vi "Is Case Selector.vi"(8 "error in":errorcluster, 11 "Terminal in":refnum<vi>) -> (0 "error out":errorcluster, 3 "Is Case Selector":bool)   [LabVIEW 2023]
doc: "Returns True is case selector is of cluaster type (as in Error Cluster)."
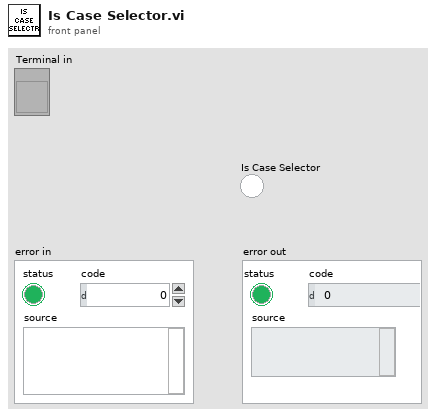
[diagram p1: front panel]
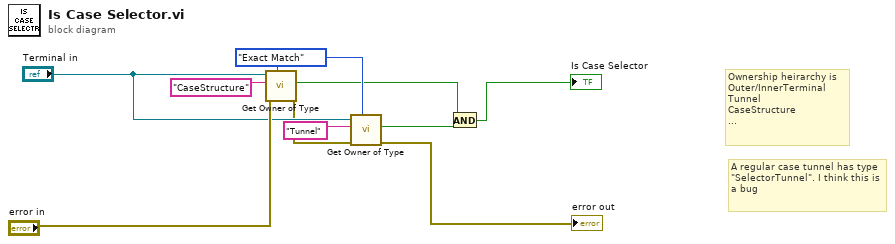
[diagram p0: block diagram]
diagram:
  w6 = enum16{"Exact Match", "Contains"}."Exact Match" ("Match Type")
  # "A regular case tunnel has type \"SelectorTunnel\". I think this is a bug"
  # "Ownership heirarchy is\nOuter/InnerTerminal\nTunnel\nCaseStructure\n..."
  n1 = call "Get Owner of Type.vi"("Match Type"=w6, "error in"="error in", "Owner Class Name desired"="CaseStructure", "reference"="Terminal in") -> ("error out"=w5:errorcluster, "Owner of type found?"=w2:bool)  [unwired: 3 in, 3 out]
  n2 = call "Get Owner of Type.vi"("Match Type"=w6, "error in"=w5, "Owner Class Name desired"="Tunnel", "reference"="Terminal in") -> ("error out"=→"error out":errorcluster, "Owner of type found?"=w3:bool)  [unwired: 3 in, 3 out]
  n3 = And(x=w2, y=w3) -> (x .and. y?=→"Is Case Selector":bool)
